vi "Check Library is Editable.vi"(8 "error in (no error)":errorcluster, 11 "LVClassLibrary in":refnum<vi>) -> (0 "error out":errorcluster, 2 "Library Editable":bool, 3 "LVClassLibrary out":refnum<vi>)   [LabVIEW 2018, in "Scripting.lvlib"]
uses:
  Scripting.lvlib
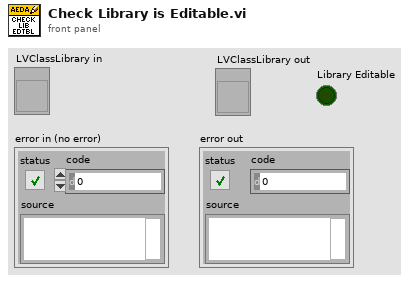
[diagram p1: front panel]
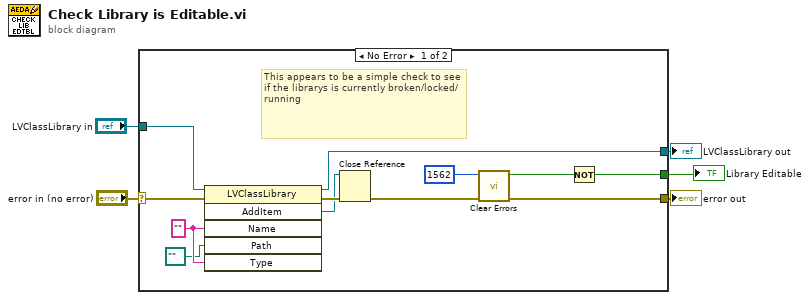
[diagram p0: block diagram]
diagram:
  n1 = case shown="No Error" "error in (no error)" {
    selector: "error in (no error)" -> [w15 w18]
    tunnel: [w8 w18] -> w5
    tunnel: "LVClassLibrary in" -> [w12 w19]
    tunnel: [w11 w19] -> w2
    tunnel: [w6 _] -> w1
    frame No Error {
      w14 = "" ("Name")
      # "This appears to be a simple check to see if the librarys is currently broken/locked/running"
      n2 = invoke class="LVClassLibrary" method="AddItem"(reference=w12, error in=w15, "Name"=w14, "Path"=path "", "Type"=w14) -> (reference out=w11:refnum<vi>, error out=w17:errorcluster, "AddItem"=w16:refnum<vi>)  [unwired: 1 in, 3 out]
      n3 = Close Reference(reference=w16, error in (no error)=w17) -> (error out=w10:errorcluster)
      n4 = call <vilib>:"Clear Errors.vi"("error in (no error)"=w10, "specific error code to clear (0: all)"=1562) -> ("error out"=w8:errorcluster, "specific error cleared?"=w7:bool)  [unwired: 4 in]
      n5 = Not(x=w7) -> (.not. x?=w6:bool)
    }
    frame Error {
    }
  }
  "error out" <- w5
  "LVClassLibrary out" <- w2
  "Library Editable" <- w1
